vi "Counter - Continuous Output.vi"() -> ()   [LabVIEW 2017]
doc: "This example demonstrates how to continuously generate digital pulses using a counter output."
uses:
  <vilib>/Utility/error.llb/DialogType.ctl
  <vilib>/DAQmx/create/channels.llb/DAQmx Create Channel (CO-Pulse Generation-Frequency).vi
  <vilib>/DAQmx/configure/timing.llb/DAQmx Timing (Implicit).vi
  <vilib>/DAQmx/configure/trigger.llb/DAQmx Start Trigger (Digital Edge).vi
  <resource>/objmgr/daqmx.rc
panel:
  out "Actual Duty Cycle":dbl
  out "Actual Frequency":dbl
  in  "Duty Cycle":dbl=0.5 format="%.6f"
  in  "Frequency (kHz)":dbl=125.0 format="%.6f"
  in  "Output Terminal":tag="/Dev1/PFI2"
  in  "Trigger Type":T1(tab)
  in  "Edge":i32(ring)=10280 items=["Rising"=10280, "Falling"=10171]
  in  "Digital Trigger Source":tag
  in  "Pause When":i32(ring)=10192 items=["High"=10192, "Low"=10214]
  in  "Pause Trigger Source":tag
  in  "Stop":bool
  in  "Counter":tag="Dev1/ctr0"
  # "Channel Settings"
  # "Trigger Settings"
  # "To configure and use a trigger you must have the necessary tab selected above."
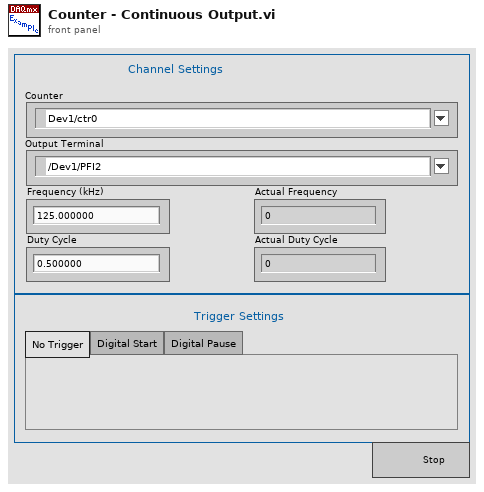
[diagram p1: front panel]
types:
  T1 = enum32{"No Trigger", "Digital Start", "Digital Pause"}
  T2 = typedef "DialogType.ctl" = u16
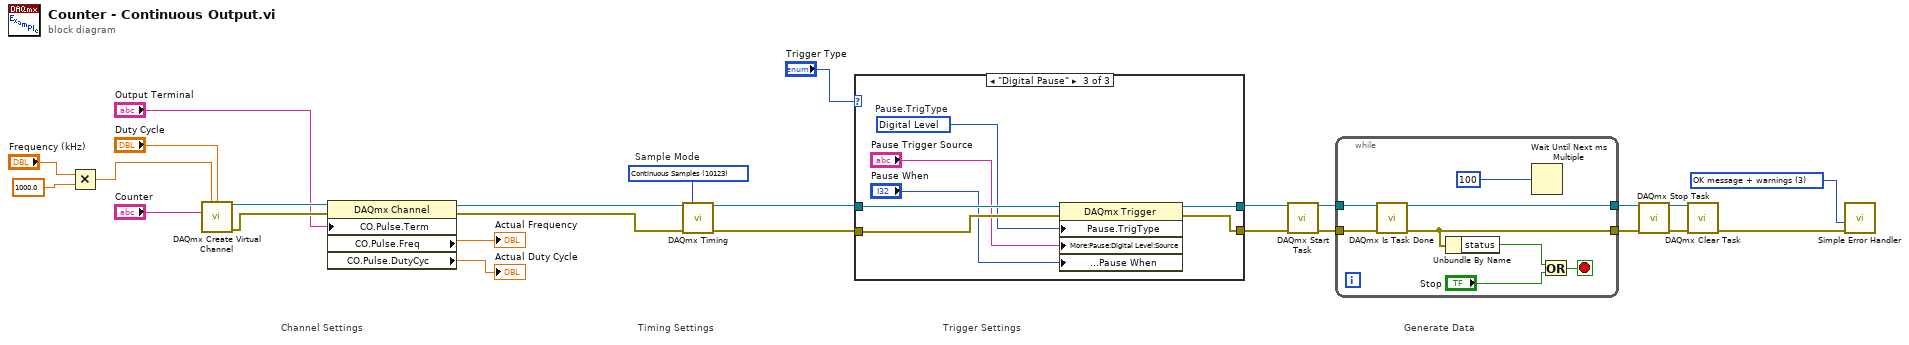
[diagram p0: block diagram]
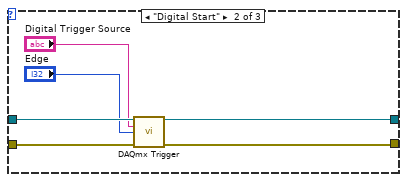
[diagram p3: hidden frame]
diagram:
  w4 = T2 3 items=["no dialog", "OK message", "continue or stop message", "OK message + warnings", "continue/stop + warnings"] ("type of dialog (OK msg:1)")
  w26 = 10123 items=["Finite Samples"=10178, "Continuous Samples"=10123, "Hardware Timed Single Point"=12522]  # Sample Mode
  # "Generate Data"
  # "Trigger Settings"
  # "Timing Settings"
  # "Channel Settings"
  n1 = Multiply(x="Frequency (kHz)", y=1000.0) -> (x*y=w1:dbl)
  n2 = call-poly <vilib>:"DAQmx Create Virtual Channel.vi"("frequency"=w1, "duty cycle"="Duty Cycle", "counter"="Counter") -> ("task out"=w16:refnum<k21>, "error out"=w15:errorcluster)  [unwired: 11 in]
  n3 = property class="DAQmx Channel"(reference=w16, error in=w15, "CO.Pulse.Term"="Output Terminal") -> (reference out=w12:refnum<k21>, error out=w13:errorcluster, "CO.Pulse.Freq"=→"Actual Frequency":dbl, "CO.Pulse.DutyCyc"=→"Actual Duty Cycle":dbl)
  n4 = call-poly <vilib>:"DAQmx Timing.vi"("task/channels in"=w12, "sample mode"=w26, "error in"=w13) -> ("task out"=w20:refnum<k21>, "error out"=w19:errorcluster)  [unwired: 11 in]
  n5 = case shown="\"Digital Pause\"" "Trigger Type" {
    tunnel: w20 -> [w28 w34 w41]
    tunnel: w19 -> [w27 w33 w38]
    tunnel: [w28 w32 w40] -> w17
    tunnel: [w27 w31 w39] -> w18
    frame "No Trigger", Default {
    }
    frame "Digital Start" {
      n6 = call-poly <vilib>:"DAQmx Trigger.vi"("task/channels in"=w34, "source"="Digital Trigger Source", "edge"="Edge", "error in"=w33) -> ("task out"=w32:refnum<k21>, "error out"=w31:errorcluster)  [unwired: 10 in]
    }
    frame "Digital Pause" {
      w37 = 10152 items=["Analog Level"=10101, "Analog Window"=10103, "Digital Level"=10152, "Digital Pattern"=10398, "None"=10230]  # Pause.TrigType
      n7 = property class="DAQmx Trigger"(reference=w41, error in=w38, "Pause.TrigType"=w37, "More:Pause:Digital Level:Source"="Pause Trigger Source", "More:Pause:Digital Level:Pause When"="Pause When") -> (reference out=w40:refnum<k21>, error out=w39:errorcluster)
    }
  }
  n8 = call <vilib>:"DAQmx Start Task.vi"("task/channels in"=w17, "error in"=w18) -> ("task out"=w25:refnum<k21>, "error out"=w24:errorcluster)  [unwired: 12 in]
  n9 = while {
    tunnel: w25 -> [w49]
    tunnel: w24 -> [w48]
    tunnel: [w45] -> w5
    tunnel: [w46] -> w6
    stop <- w47 stop-if-true
    n10 = call <vilib>:"DAQmx Is Task Done.vi"("task/channels in"=w49, "error in"=w48) -> ("task out"=w46:refnum<k21>, "error out"=w45:errorcluster)  [unwired: 11 in, 1 out]
    n11 = Unbundle By Name(w45) -> ("status"=w44:bool)
    n12 = Wait Until Next ms Multiple(millisecond multiple=u32 100) -> ()  [unwired: 1 out]
    n13 = Or(x=w44, y="Stop") -> (x .or. y?=w47:bool)
  }
  n14 = call <vilib>:"DAQmx Stop Task.vi"("task/channels in"=w6, "error in"=w5) -> ("task out"=w8:refnum<k21>, "error out"=w7:errorcluster)  [unwired: 12 in]
  n15 = call <vilib>:"DAQmx Clear Task.vi"("task in"=w8, "error in"=w7) -> ("error out"=w23:errorcluster)  [unwired: 13 in]
  n16 = call <vilib>:"Simple Error Handler.vi"("type of dialog (OK msg:1)"=w4, "error in (no error)"=w23) -> ()  [unwired: 3 in, 5 out]
